vi "Resize and Align Image based on Change in dimensions and midpoint.vi"(9 "Modified X Mid point Pixel (After Non-Linear Stretch)":i32, 10 "Initial Dimension (1D Array: Ypxls,XPxls)":i32[](array[numeric]), 11 "Modified Image Array (2D)":u8[][](array[numeric])) -> (3 "Resized-Recentered Image Array (2D)":u8[][](array[numeric]))   [LabVIEW 2012]
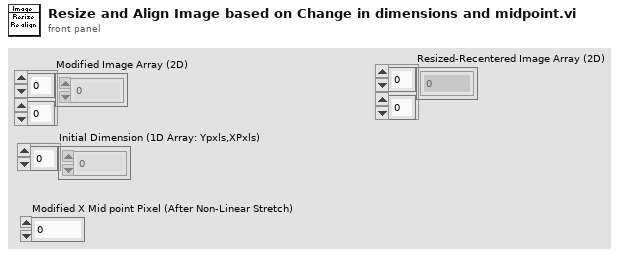
[diagram p1: front panel]
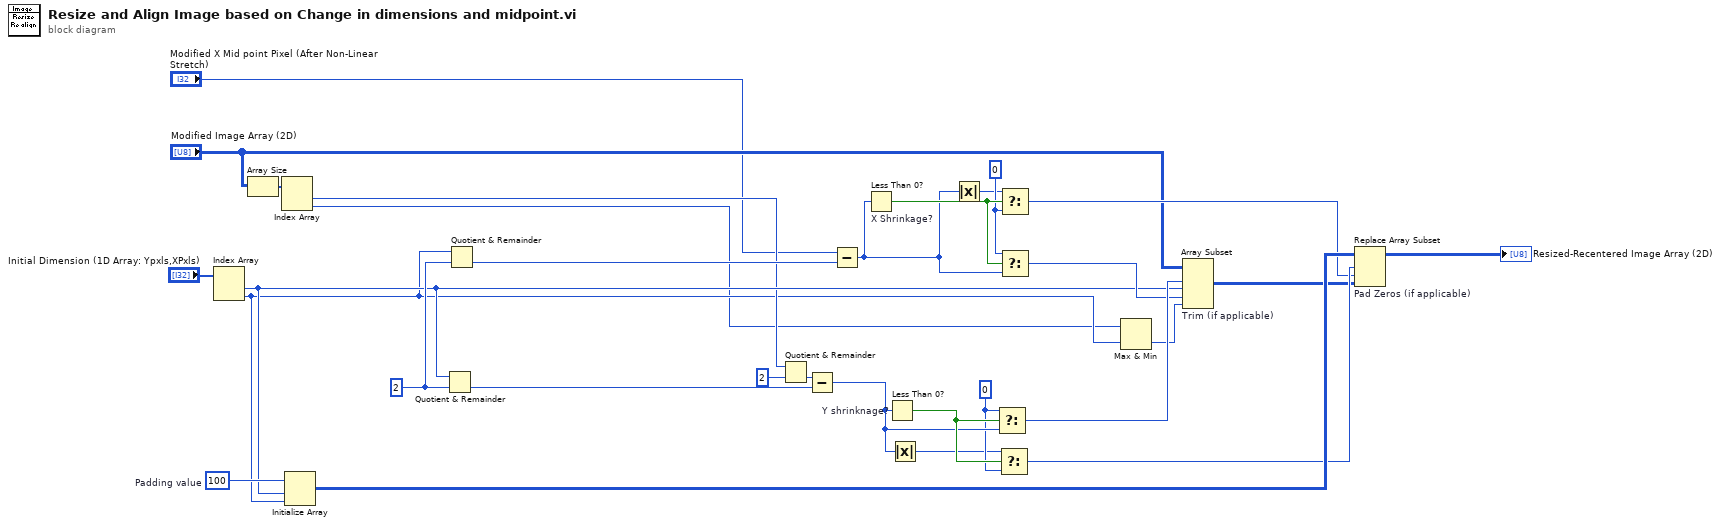
[diagram p0: block diagram]
diagram:
  w18 = 2 ("y")
  w21 = 0 ("x-y")
  w22 = 0 ("x-y")
  w30 = u8 100  # Padding value
  n1 = Index Array(array="Initial Dimension (1D Array: Ypxls,XPxls)") -> (element #1=w15:i32, element #2=w9:i32)  [unwired: 2 in]
  n2 = Array Size(array="Modified Image Array (2D)") -> (size(s)=w19:i32[])
  n3 = Index Array(array=w19) -> (element #1=w14:i32, element #2=w5:i32)  [unwired: 2 in]
  n4 = Initialize Array(w30, w15, w9) -> (w27:u8[][])
  n5 = Quotient & Remainder(x=w15, y=w18) -> (floor(x/y)=w17:i32)  [unwired: 1 out]
  n6 = Quotient & Remainder(x=w9, y=w18) -> (floor(x/y)=w16:i32)  [unwired: 1 out]
  n7 = Quotient & Remainder(x=w14, y=2) -> (floor(x/y)=w12:i32)  [unwired: 1 out]
  n8 = Subtract(x=w12, y=w17) -> (x-y=w23:i32)
  n9 = Subtract(x="Modified X Mid point Pixel (After Non-Linear Stretch)", y=w16) -> (x-y=w25:i32)
  n10 = Less Than 0? "X Shrinkage?"(x=w25) -> (x < 0?=w26:bool)
  n11 = Less Than 0? "Y shrinknage?"(x=w23) -> (x < 0?=w24:bool)
  n12 = Absolute Value(x=w23) -> (abs(x)=w11:i32)
  n13 = Absolute Value(x=w25) -> (abs(x)=w10:i32)
  n14 = Select(t=w22, s=w24, f=w23) -> (s? t:f=w29:i32)
  n15 = Select(t=w11, s=w24, f=w22) -> (s? t:f=w20:i32)
  n16 = Select(t=w10, s=w26, f=w21) -> (s? t:f=w8:i32)
  n17 = Select(t=w21, s=w26, f=w25) -> (s? t:f=w28:i32)
  n18 = Max & Min(x=w5, y=w9) -> (min(x,y)=w7:i32)  [unwired: 1 out]
  n19 = Array Subset "Trim (if applicable)"(array="Modified Image Array (2D)", index (row)=w29, length (row)=w15, index (col)=w28, length (col)=w7) -> (w6:u8[][])
  n20 = Replace Array Subset "Pad Zeros (if applicable)"(array=w27, new element=w6, index (row)=w20, index (col)=w8) -> (→"Resized-Recentered Image Array (2D)":u8[][])
